vi "CalcTrms.vi"(6 "CAMpos":u16, 7 "TRMSpix":u32, 8 "error in (no error)":errorcluster, 9 "lastSample":u32, 10 "firstSample":u32) -> (0 "error out":errorcluster, 1 "TRMS 2":dbl=255.0, 2 "mean 2":dbl=255.0, 3 "TRMS 1":dbl=255.0, 5 "mean 1":dbl=255.0)   [LabVIEW 2015, in "ESLSCDLL.lvlib"]
uses:
  ESLSCDLL.lvlib
  Globals.vi
  ESLSCDLL.dll
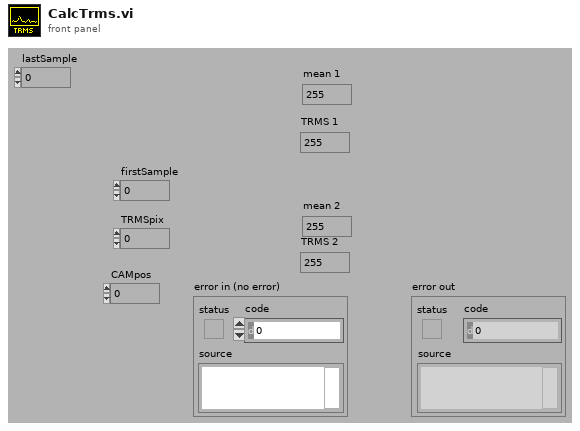
[diagram p1: front panel]
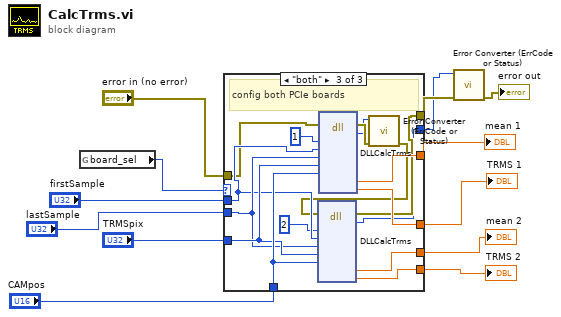
[diagram p0: block diagram]
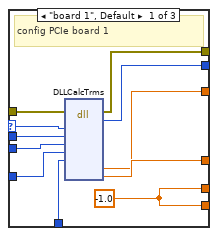
[diagram p2: hidden frame]
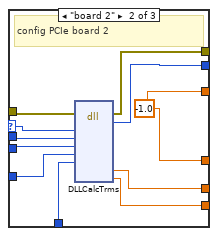
[diagram p3: hidden frame]
diagram:
  n1 = global read "Globals.vi" "board_sel"() -> (w1:enum32{"0", "board 1", "board 2", "both"})
  n2 = case shown="\"both\"" w1 {
    selector: w1 -> [w24 w34 _]
    tunnel: "TRMSpix" -> [w22 w31 w49]
    tunnel: [w19 w28 w42] -> w12
    tunnel: "firstSample" -> [w23 w33 w47]
    tunnel: [w21 w35 w44] -> w10
    tunnel: [w20 w35 w45] -> w9
    tunnel: [w19 w29 w43] -> w8
    tunnel: "CAMpos" -> [w18 w30 w50]
    tunnel: "lastSample" -> [w17 w32 w48]
    tunnel: "error in (no error)" -> [w16 w27 w41]
    tunnel: [w15 w26 w37] -> w3
    tunnel: [w14 w25 w36] -> w2
    frame "board 1", Default {
      w19 = -1.0
      # "config PCIe board 1"
      n3 = dll-call lib="C:/ENTW/PCIE/LV64/board.vis/ESLSCDLL.dll" fn="DLLCalcTrms" ("lwlscdll.dll:DLLReadLongS0")(error in=w16, "drv"=w24, "firstSample"=w23, "lastSample"=w17, "TRMSpix"=w22, "CAMpos"=w18) -> (error out=w15:errorcluster, "es_status_codes"=w14:i32, "mwf"=w20:dbl, "trms"=w21:dbl)  [unwired: 9 in, 1 out]
    }
    frame "board 2" {
      w35 = -1.0
      # "config PCIe board 2"
      n4 = dll-call lib="C:/ENTW/PCIE/LV64/board.vis/ESLSCDLL.dll" fn="DLLCalcTrms" ("lwlscdll.dll:DLLReadLongS0")(error in=w27, "drv"=w34, "firstSample"=w33, "lastSample"=w32, "TRMSpix"=w31, "CAMpos"=w30) -> (error out=w26:errorcluster, "es_status_codes"=w25:i32, "mwf"=w29:dbl, "trms"=w28:dbl)  [unwired: 9 in, 1 out]
    }
    frame "both" {
      # "config both PCIe boards"
      n5 = dll-call lib="C:/ENTW/PCIE/LV64/board.vis/ESLSCDLL.dll" fn="DLLCalcTrms" ("lwlscdll.dll:DLLReadLongS0")(error in=w41, "drv"=u32 1, "firstSample"=w47, "lastSample"=w48, "TRMSpix"=w49, "CAMpos"=w50) -> (error out=w40:errorcluster, "es_status_codes"=w39:i32, "mwf"=w45:dbl, "trms"=w44:dbl)  [unwired: 9 in, 1 out]
      n6 = call "Error Converter (ErrCode or Status).vi"("error in (no error)"=w40, "error code"=w39) -> ("error out"=w38:errorcluster)  [unwired: 9 in]
      n7 = dll-call lib="C:/ENTW/PCIE/LV64/board.vis/ESLSCDLL.dll" fn="DLLCalcTrms" ("lwlscdll.dll:DLLReadLongS0")(error in=w38, "drv"=u32 2, "firstSample"=w47, "lastSample"=w48, "TRMSpix"=w49, "CAMpos"=w50) -> (error out=w37:errorcluster, "es_status_codes"=w36:i32, "mwf"=w43:dbl, "trms"=w42:dbl)  [unwired: 9 in, 1 out]
    }
  }
  "TRMS 1" <- w10
  "TRMS 2" <- w12
  "mean 1" <- w9
  "mean 2" <- w8
  n8 = call "Error Converter (ErrCode or Status).vi"("error in (no error)"=w3, "error code"=w2) -> ("error out"=→"error out":errorcluster)  [unwired: 9 in]
